vi "CTL_TestPV.vi"(4 "Level B":dbl=8.5 format="%#_13g", 6 "Level M":dbl=-0.6 format="%#_13g", 9 "Level SP in":dbl) -> (2 "Level Sense":dbl, 3 "PV Level Inch":dbl)   [LabVIEW 2024]
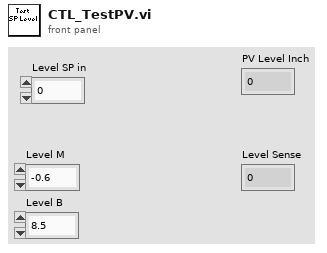
[diagram p1: front panel]
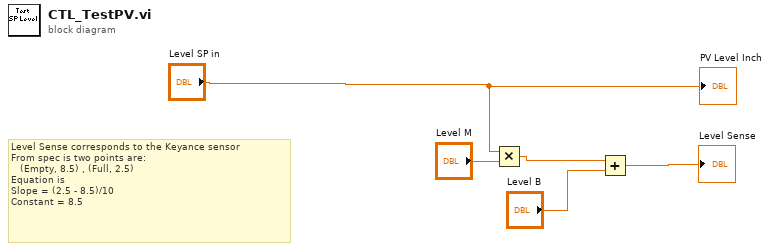
[diagram p0: block diagram]
diagram:
  # "Level Sense corresponds to the Keyance sensor\nFrom spec is two points are:\n   (Empty, 8.5) , (Full, 2.5)\nEquation is \nSlope = (2.5 - 8.5)/10\nConstant = 8.5"
  n1 = Multiply(x="Level SP in", y="Level M") -> (x*y=w5:dbl)
  n2 = Add(x=w5, y="Level B") -> (x+y=→"Level Sense":dbl)
  "PV Level Inch" <- "Level SP in"
